vi "Write to OPC Server.vi"() -> ()   [LabVIEW 2015]
panel:
  out "OPC URL":string
  in  "Stop Button":bool
  in  "Numeric Control":dbl=22.0
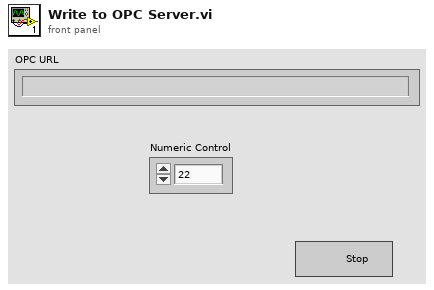
[diagram p1: front panel]
types:
  T1 = enum16{"Read", "Write", "ReadWrite", "BufferedRead", "BufferedReadWrite"}
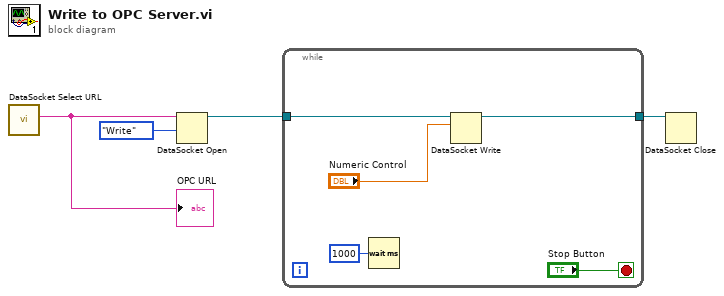
[diagram p0: block diagram]
diagram:
  n1 = call <vilib>:"DataSocket Select URL.vi"() -> ("URL"=w1:string)  [unwired: 9 in, 2 out]
  "OPC URL" <- w1
  n2 = DataSocket Open(10:T1."Write" ("mode"), 11:w1) -> (3:w4:refnum<k13>)  [unwired: 2 in, 1 out]
  n3 = while {
    tunnel: w4 -> [w7]
    tunnel: [w6] -> w3
    stop <- "Stop Button" stop-if-true
    n4 = Wait (ms)(milliseconds to wait=u32 1000) -> ()  [unwired: 1 out]
    n5 = DataSocket Write(10:"Numeric Control", 11:w7) -> (3:w6:refnum<k13>)  [unwired: 2 in, 2 out]
  }
  n6 = DataSocket Close(11:w3) -> ()  [unwired: 2 in, 2 out]
